vi "create.vi"(7 "ID":string, 8 "error in (no error)":errorcluster, 10 "name":string, 11 "XMLElement in":refnum<class "XMLElement.lvclass">) -> (0 "error out":errorcluster, 3 "XMLElement out":refnum<class "XMLElement.lvclass">)   [LabVIEW 2010, in "XMLElement.lvclass"]
uses:
  XMLElement.lvclass
  XMLElement.lvclass/XMLElement.ctl
  <vilib>/xml/NI_XML.lvlib
  Program Files/National Instruments/LabVIEW 2010/resource/objmgr/DOMUserDefRef.rc
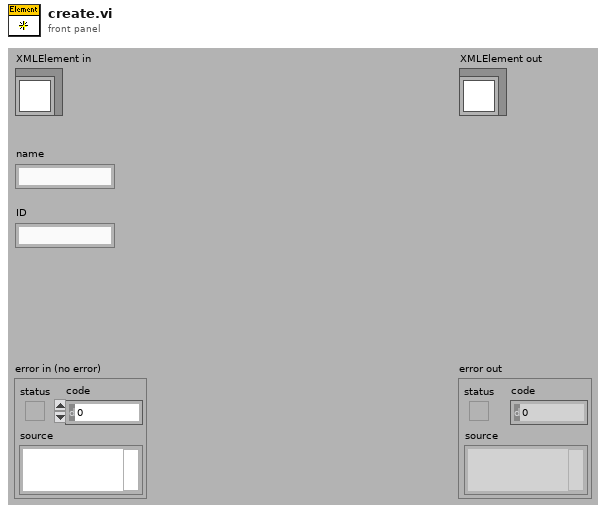
[diagram p1: front panel]
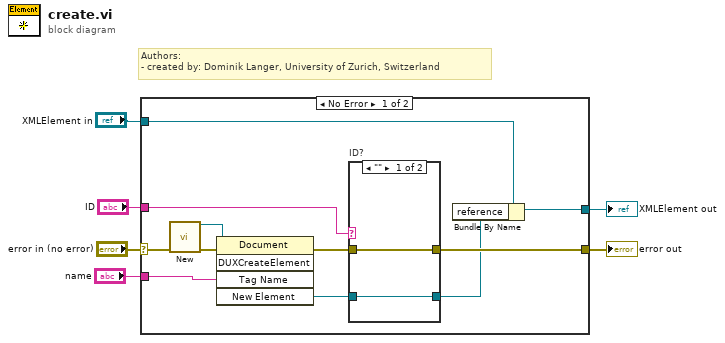
[diagram p0: block diagram]
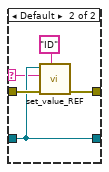
[diagram p2: hidden frame]
diagram:
  # "Authors: \n- created by: Dominik Langer, University of Zurich, Switzerland"
  n1 = case shown="No Error" "error in (no error)" {
    selector: "error in (no error)" -> [w17 w26]
    tunnel: [w12 w26] -> w5
    tunnel: [w7 w25] -> w3
    tunnel: "XMLElement in" -> [w8 w25]
    tunnel: "name" -> [w14 _]
    tunnel: "ID" -> [w10 _]
    frame No Error {
      n2 = call <vilib>:"New.vi"("error in (no error)"=w17) -> ("error out"=w16:errorcluster, "DOM document out"=w15:refnum<k20>)  [unwired: 7 in]
      n3 = invoke class="Document" method="DUXCreateElement"(reference=w15, error in=w16, "Tag Name"=w14) -> (error out=w13:errorcluster, "New Element"=w11:refnum<k20>)  [unwired: 2 in, 3 out]
      n4 = case "ID?" shown="\"\"" w10 {
        selector: w10 -> [_ w20]
        tunnel: w13 -> [w19 w24]
        tunnel: [w19 w23] -> w12
        tunnel: w11 -> [w18 w22]
        tunnel: [w18 w22] -> w9
        frame "" {
        }
        frame Default {
          n5 = call "set_value_REF.vi"("attribute name"="ID", "error in (no error)"=w24, "value"=w20, "Element ref in"=w22) -> ("error out"=w23:errorcluster)  [unwired: 6 in, 1 out]
        }
      }
      n6 = Bundle By Name(cluster=w8, "reference"=w9) -> (w7:refnum<class "XMLElement.lvclass">)
    }
    frame Error {
    }
  }
  "error out" <- w5
  "XMLElement out" <- w3
